vi "Write Report Interface.vi"(8 "error in (no error)":errorcluster, 10 "Report Interface":refnum<class "Report Interface.lvclass">, 11 "Report Generator in":refnum<class "Report Generator.lvclass">) -> (0 "error out":errorcluster, 3 "Report Generator out":refnum<class "Report Generator.lvclass">)   [LabVIEW 2020, in "Reports.lvlib" / "Report Generator.lvclass"]
uses:
  Report Generator.lvclass
  Framework/Report Interface/Report Interface.lvclass
  Report Generator.lvclass/Report Generator.ctl
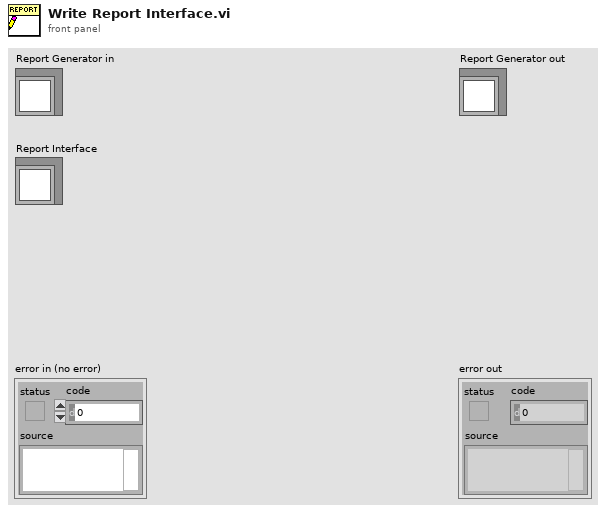
[diagram p1: front panel]
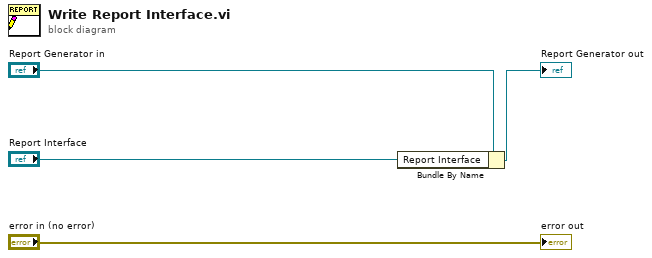
[diagram p0: block diagram]
diagram:
  n1 = Bundle By Name(cluster="Report Generator in", "Report Interface"="Report Interface") -> (→"Report Generator out":refnum<class "Report Generator.lvclass">)
  "error out" <- "error in (no error)"
